vi "Comemso BCS Mngr.vi"(7 "Action":T4, 8 "error in (no error)":errorcluster, 11 "Data in":T3[](array[typedef])) -> (0 "error out":errorcluster, 2 "data":dbl[](array[numeric]) format="%.2f", 3 "Data out":T3[](array[typedef]))   [LabVIEW 2021]
uses:
  <vilib>/xnet/xnet.llb/XNET Create Session (Signal Input Single-point).vi
  <resource>/objmgr/xnet.rc
  <vilib>/xnet/xnet.llb/XNET Read (Signal Single-point).vi
  <vilib>/xnet/xnet.llb/XNET Create Session (Frame Input Stream).vi
  <vilib>/xnet/xnet.llb/XNET Write (Frame CAN).vi
  <vilib>/xnet/xnet.llb/XNET Create Session (Frame Output Single-point).vi
  <vilib>/xnet/xnet.llb/XNET Write (Signal Single-point).vi
  <vilib>/xnet/xnet.llb/XNET Create Session (Signal Output Single-point).vi
  <vilib>/xnet/xnet.llb/XNET Create Session (Conversion).vi
  <vilib>/xnet/xnet.llb/XNET Read (Frame CAN).vi
  <vilib>/xnet/xnet.llb/XNET Convert (Signal to Frame CAN).vi
  <vilib>/xnet/xnet.llb/XNET Create Session (Frame Input Single-point).vi
  controls/BCS Manager.ctl
  controls/Signal Data.ctl
  controls/CANbus com type.ctl
  controls/Transfer Type.ctl
panel:
  in  "timeout":i32=-1
  in  "Data Type":T1
  in  "Read Type":T2
  in  "number to read":i32=-1
  in  "database alias":string="Database"
  in  "interface":refnum<k21>="CAN1"
  in  "Termination":u32(ring) items=["Off", "On"]
  in  "Baud Rate":u64=1000000
  in  "filepath":path=path "C:/Users/ykouchnir/Desktop/Comemso BCS Tester/BCS24_CAN-MatrixV7_12.dbc"
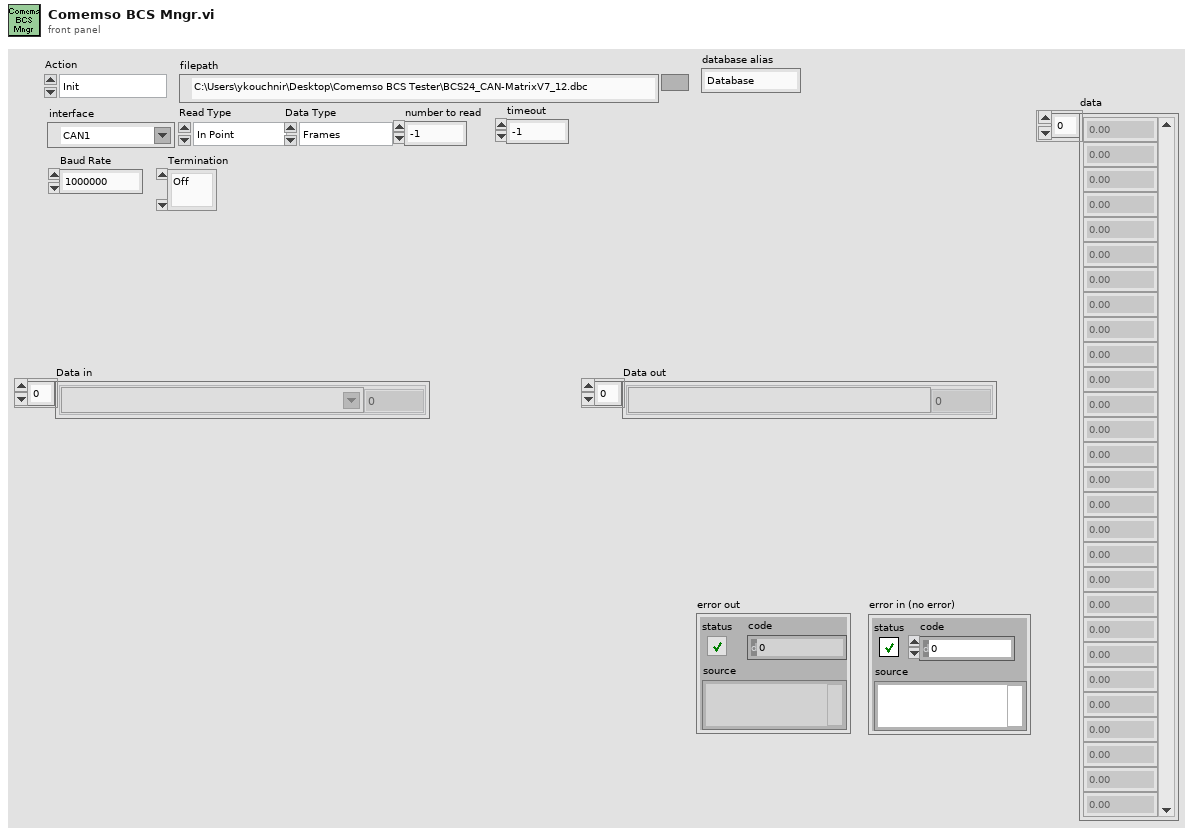
[diagram p1: front panel]
types:
  T1 = typedef "Transfer Type.ctl" = enum16{"Frames", "Signals"}
  T2 = typedef "CANbus com type.ctl" = enum16{"In Point", "Queued", "Stream"}
  T3 = typedef "Signal Data.ctl" = cluster{"XNET Signal":refnum<k21>, "Data":dbl}
  T4 = typedef "BCS Manager.ctl" = enum16{"Init", "Start Signal Session", "Start Frame Session", "Write Sigs Session", "Write Frames Session", "Write Sigs Single", "Write Frames Single", "Read Sigs Session", "Read Frames Session", "Read Sigs Single", "Read Frames Single", "Write Raw Frame Session", "Write Raw Frame Single", "FrameRef to Sigs", "FrameID to FrameRef", "Close"}
  T5 = typedef "XNET Frame CAN.ctl" = cluster{"timestamp":timestamp, "payload":u8[], "identifier":u32, "type":T6, "extended?":bool, "echo?":bool}
  T6 = typedef "XNET Frame Type CAN.ctl" = u8
  T7 = typedef "Frame Data.ctl" = cluster{"Raw Frame":T5, "Frame Name":refnum<k21>, "Signals":T3[]}
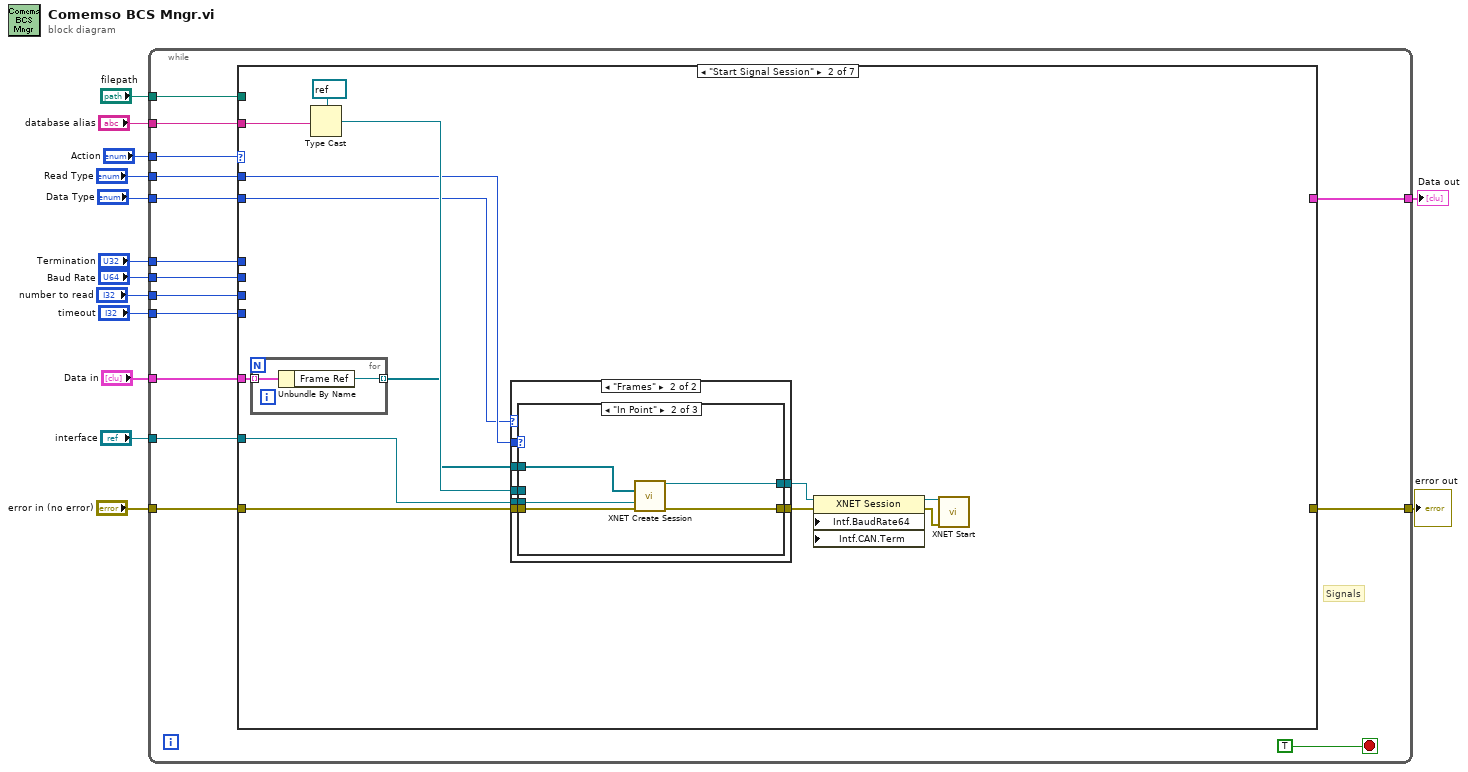
[diagram p0: block diagram]
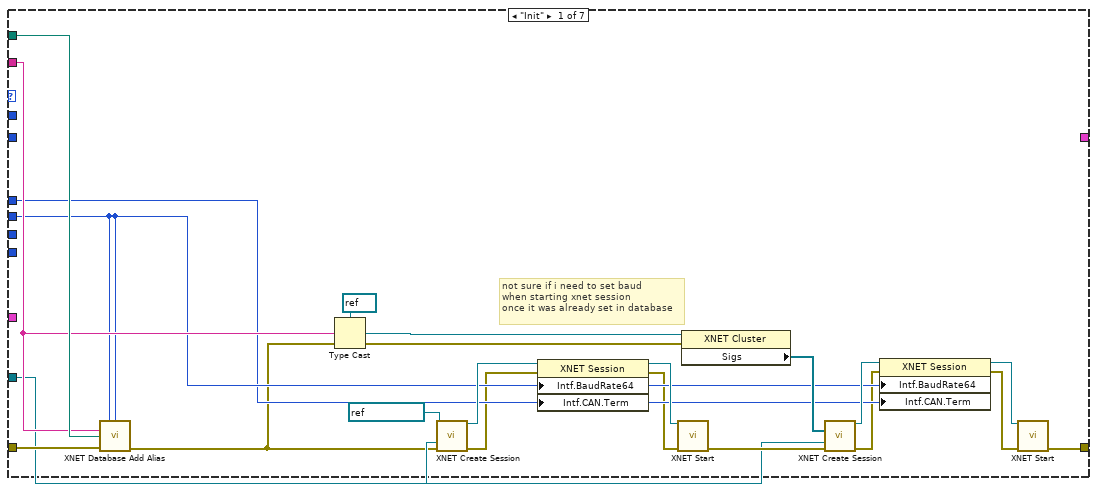
[diagram p2: hidden frame]
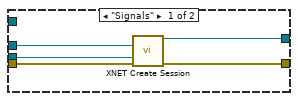
[diagram p3: hidden frame]
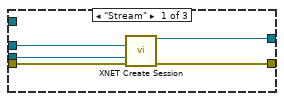
[diagram p4: hidden frame]
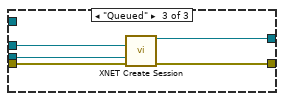
[diagram p5: hidden frame]
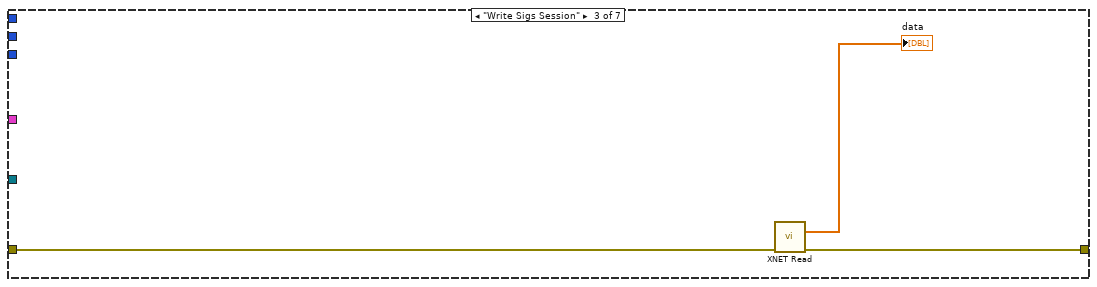
[diagram p6: hidden frame]
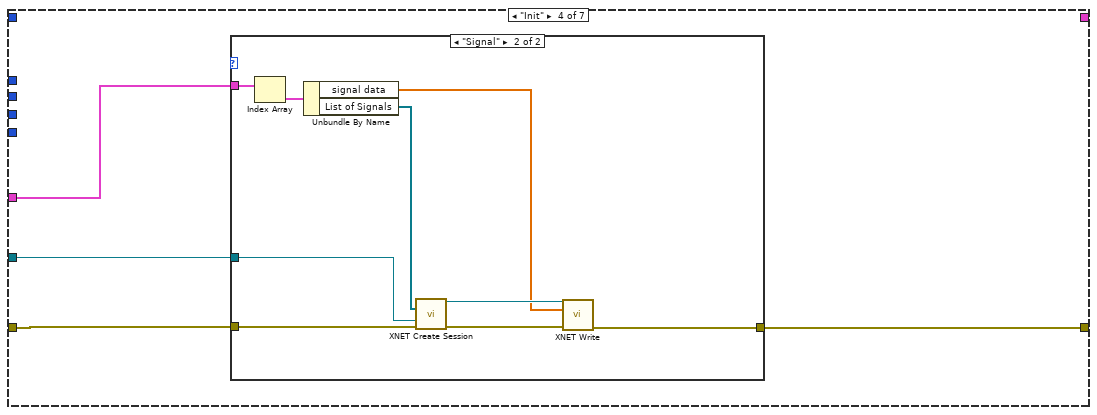
[diagram p7: hidden frame]
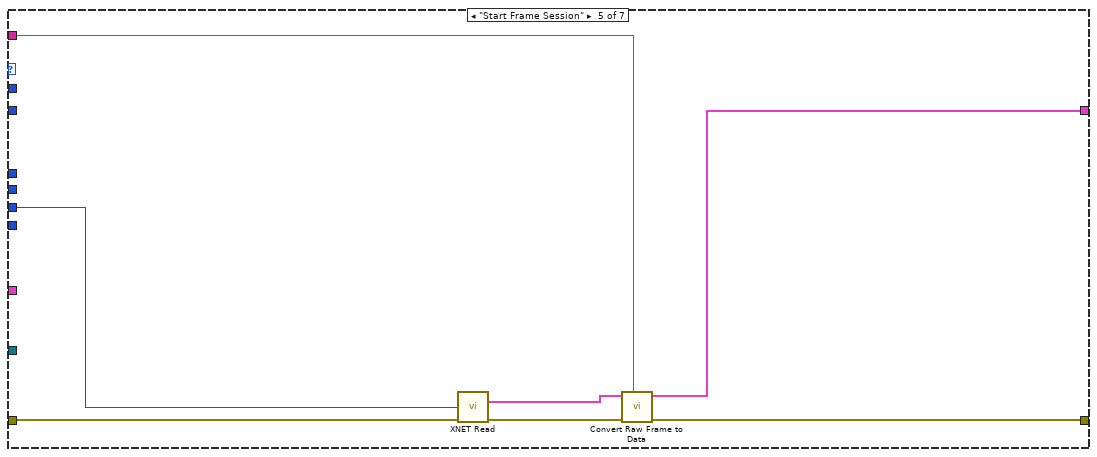
[diagram p9: hidden frame]
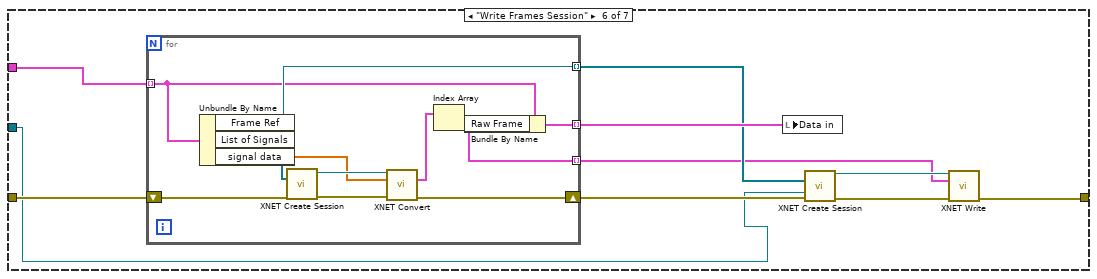
[diagram p10: hidden frame]
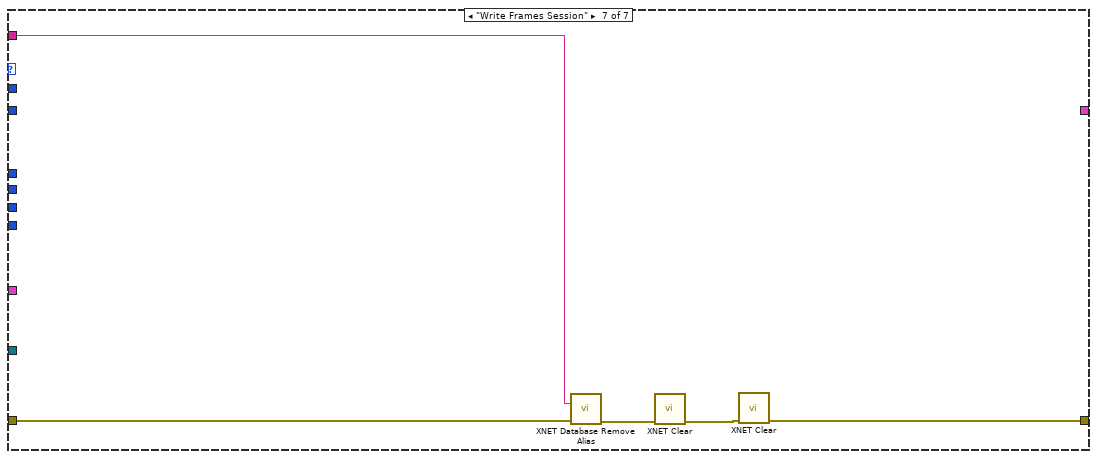
[diagram p11: hidden frame]
diagram:
  n1 = while {
    tunnel: "Action" -> [w28]
    tunnel: "error in (no error)" -> [w27]
    tunnel: "filepath" -> [w26]
    tunnel: [w25] -> w11
    tunnel: "Baud Rate" -> [w24]
    tunnel: "Termination" -> [w23]
    tunnel: "interface" -> [w22]
    tunnel: "database alias" -> [w21]
    tunnel: [w20] -> w6
    tunnel: "Data in" -> [w19]
    tunnel: "Data Type" -> [w18]
    tunnel: "Read Type" -> [w17]
    tunnel: "number to read" -> [w16]
    tunnel: "timeout" -> [w15]
    stop <- TRUE stop-if-true
    # "Signals"
    n2 = case shown="\"Start Signal Session\"" w28 {
      tunnel: w27 -> [w50 w60 w94 w99 w114 w123 w141]
      tunnel: w26 -> [w49 _ _ _ _ _ _]
      tunnel: [w40 _ w95 w98 w115 w117 w138] -> w25
      tunnel: w24 -> [w37 _ _ _ _ _ _]
      tunnel: w23 -> [w36 _ _ _ _ _ _]
      tunnel: w22 -> [w43 w51 _ w97 _ w118 _]
      tunnel: w21 -> [w46 w62 _ _ w110 _ w137]
      tunnel: [_ _ _ _ w111 _ _] -> w20
      tunnel: w19 -> [_ w55 _ w96 _ w125 _]
      tunnel: w18 -> [_ w52 _ _ _ _ _]
      tunnel: w17 -> [_ w53 _ _ _ _ _]
      tunnel: w16 -> [_ _ _ _ w109 _ _]
      tunnel: w15 -> [_ _ _ _ _ _ _]
      frame "Init" {
        # "not sure if i need to set baud \nwhen starting xnet session\nonce it was already set in database"
        n3 = call <vilib>:"XNET Database Add Alias.vi"("default baud rate (0)"=w37, "default FD baud rate (0)"=w37, "alias"=w46, "filepath"=w49, "error in (no error)"=w50) -> ("error out"=w30:errorcluster)  [unwired: 10 in]
        n4 = Type Cast(type=refnum<k21> refnum ("cluster (:memory:)"), x=w46) -> (*(type *) &x=w42:refnum<k21>)
        n5 = call-poly <vilib>:"XNET Create Session.vi"("cluster (:memory:)"=refnum<k21> "Database", "interface"=w43, "error in (no error)"=w30) -> ("session out"=w48:refnum<k21>, "error out"=w34:errorcluster)  [unwired: 11 in]
        n6 = property class="XNET Session"(reference=w48, error in=w34, "Intf.BaudRate64"=w37, "Intf.CAN.Term"=w36) -> (reference out=w47:refnum<k21>, error out=w33:errorcluster)
        n7 = call <vilib>:"XNET Start.vi"("session in"=w47, "error in (no error)"=w33) -> ("error out"=w44:errorcluster)  [unwired: 12 in, 1 out]
        n8 = property class="XNET Cluster"(reference=w42, error in=w30) -> ("Sigs"=w41:refnum<k21>[])  [unwired: 2 out]
        n9 = call-poly <vilib>:"XNET Create Session.vi"("signal list"=w41, "interface"=w43, "error in (no error)"=w44) -> ("session out"=w39:refnum<k21>, "error out"=w32:errorcluster)  [unwired: 11 in]
        n10 = property class="XNET Session"(reference=w39, error in=w32, "Intf.BaudRate64"=w37, "Intf.CAN.Term"=w36) -> (reference out=w38:refnum<k21>, error out=w31:errorcluster)
        n11 = call <vilib>:"XNET Start.vi"("session in"=w38, "error in (no error)"=w31) -> ("error out"=w40:errorcluster)  [unwired: 12 in, 1 out]
      }
      frame "Start Signal Session" {
        n12 = for {
          tunnel: w55 -> [w65] mode=indexing
          tunnel: [w64] -> w54 mode=indexing
          n13 = Unbundle By Name(w65) -> ("Frame Ref"=w64:refnum<k21>)
        }
        n14 = Type Cast(type=refnum<k21> refnum ("cluster (:memory:)"), x=w62) -> (*(type *) &x=w61:refnum<k21>)
        n15 = case shown="\"Frames\"" w52 {
          tunnel: w51 -> [w70 w77]
          tunnel: w61 -> [w69 w76]
          tunnel: w60 -> [w68 w75]
          tunnel: [w67 w74] -> w59
          tunnel: [w66 w73] -> w57
          tunnel: w53 -> [_ w72]
          tunnel: w54 -> [_ w71]
          frame "Signals" {
            n16 = call-poly <vilib>:"XNET Create Session.vi"("cluster (:memory:)"=w69, "interface"=w70, "error in (no error)"=w68) -> ("session out"=w67:refnum<k21>, "error out"=w66:errorcluster)  [unwired: 11 in]
          }
          frame "Frames" {
            n17 = case shown="\"In Point\"" w72 {
              tunnel: w77 -> [w82 w87 w92]
              tunnel: w76 -> [w81 _ w91]
              tunnel: w75 -> [w80 w86 w90]
              tunnel: [w79 w85 w89] -> w74
              tunnel: [w78 w84 w88] -> w73
              tunnel: w71 -> [_ w83 _]
              frame "Stream" {
                n18 = call-poly <vilib>:"XNET Create Session.vi"("cluster (:memory:)"=w81, "interface"=w82, "error in (no error)"=w80) -> ("session out"=w79:refnum<k21>, "error out"=w78:errorcluster)  [unwired: 11 in]
              }
              frame "In Point" {
                n19 = call-poly <vilib>:"XNET Create Session.vi"("frame list"=w83, "interface"=w87, "error in (no error)"=w86) -> ("session out"=w85:refnum<k21>, "error out"=w84:errorcluster)  [unwired: 11 in]
              }
              frame "Queued" {
                n20 = call-poly <vilib>:"XNET Create Session.vi"("cluster (:memory:)"=w91, "interface"=w92, "error in (no error)"=w90) -> ("session out"=w89:refnum<k21>, "error out"=w88:errorcluster)  [unwired: 11 in]
              }
            }
          }
        }
        n21 = property class="XNET Session" props=["Intf.BaudRate64", "Intf.CAN.Term"](reference=w59, error in=w57) -> (reference out=w58:refnum<k21>, error out=w56:errorcluster)  [unwired: 2 in]
        n22 = call <vilib>:"XNET Start.vi"("session in"=w58, "error in (no error)"=w56) -> ()  [unwired: 12 in, 2 out]
      }
      frame "Write Sigs Session" {
        n23 = call-poly <vilib>:"XNET Read.vi"("error in (no error)"=w94) -> ("data"=→"data":dbl[], "error out"=w95:errorcluster)  [unwired: 12 in, 1 out]
      }
      frame "Init" {
        n24 = case shown="\"Signal\"" {
          selector: _ -> [_ _]
          tunnel: w99 -> [_ w106]
          tunnel: [_ w105] -> w98
          tunnel: w97 -> [_ w104]
          tunnel: w96 -> [_ w103]
          frame "Frame", Default {
          }
          frame "Signal" {
            n25 = Index Array(array=w103) -> (element=w102:T3)  [unwired: 1 in]
            n26 = Unbundle By Name(w102) -> ("signal data"=w101:dbl[], "List of Signals"=w100:refnum<k21>[])
            n27 = call-poly <vilib>:"XNET Create Session.vi"("signal list"=w100, "interface"=w104, "error in (no error)"=w106) -> ("session out"=w108:refnum<k21>, "error out"=w107:errorcluster)  [unwired: 11 in]
            n28 = call-poly <vilib>:"XNET Write.vi"("session in"=w108, "data"=w101, "error in (no error)"=w107) -> ("error out"=w105:errorcluster)  [unwired: 11 in, 1 out]
          }
        }
      }
      frame "Start Frame Session" {
        n29 = call-poly <vilib>:"XNET Read.vi"("number to read (-1)"=w109, "error in (no error)"=w114) -> ("data"=w112:T5[], "error out"=w113:errorcluster)  [unwired: 10 in, 2 out]
        n30 = call "Convert Raw Frame to Data.vi"("Database alias"=w110, "error in (no error)"=w113, "Raw Frames"=w112) -> ("error out"=w115:errorcluster, "Frame Data"=w111:T7[])  [unwired: 7 in]
      }
      frame "Write Frames Session" {
        n31 = for {
          shift-right: [w130] -> w121
          shift-left: w123 -> [w133]
          tunnel: w125 -> [w129] mode=indexing
          tunnel: [w134] -> w119 mode=indexing
          tunnel: [w127] -> w122 mode=indexing
          tunnel: [w126] -> w116 mode=indexing
          n32 = Unbundle By Name(w129) -> ("Frame Ref"=w134:refnum<k21>, "List of Signals"=w132:refnum<k21>[], "signal data"=w131:dbl[])
          n33 = call-poly <vilib>:"XNET Create Session.vi"("signal list"=w132, "error in (no error)"=w133) -> ("session out"=w135:refnum<k21>, "error out"=w136:errorcluster)  [unwired: 12 in]
          n34 = call-poly <vilib>:"XNET Convert.vi"("session in"=w135, "signal data"=w131, "error in (no error)"=w136) -> ("frame data"=w128:T5[], "error out"=w130:errorcluster)  [unwired: 9 in, 2 out]
          n35 = Index Array(array=w128) -> (element=w126:T5)  [unwired: 1 in]
          n36 = Bundle By Name(cluster=w129, "Raw Frame"=w126) -> (w127:T3)
        }
        n37 = local write "Data in"(w122) -> ()
        n38 = call-poly <vilib>:"XNET Create Session.vi"("frame list"=w119, "interface"=w118, "error in (no error)"=w121) -> ("session out"=w120:refnum<k21>, "error out"=w124:errorcluster)  [unwired: 11 in]
        n39 = call-poly <vilib>:"XNET Write.vi"("session in"=w120, "data"=w116, "error in (no error)"=w124) -> ("error out"=w117:errorcluster)  [unwired: 11 in, 1 out]
      }
      frame "Write Frames Session" {
        n40 = call <vilib>:"XNET Database Remove Alias.vi"("alias"=w137, "error in (no error)"=w141) -> ("error out"=w140:errorcluster)  [unwired: 13 in]
        n41 = call <vilib>:"XNET Clear.vi"("error in (no error)"=w140) -> ("error out"=w139:errorcluster)  [unwired: 14 in]
        n42 = call <vilib>:"XNET Clear.vi"("error in (no error)"=w139) -> ("error out"=w138:errorcluster)  [unwired: 14 in]
      }
    }
  }
  "error out" <- w11
  "Data out" <- w6
